vi "cook.vi"(8 "error in (no error)":errorcluster, 11 "Barbecue in":refnum<class "Barbecue.lvclass">) -> (0 "error out":errorcluster, 3 "Barbecue out":refnum<class "Barbecue.lvclass">)   [LabVIEW 2011, in "CookBehaviors.lvlib" / "Barbecue.lvclass"]
uses:
  Barbecue.lvclass
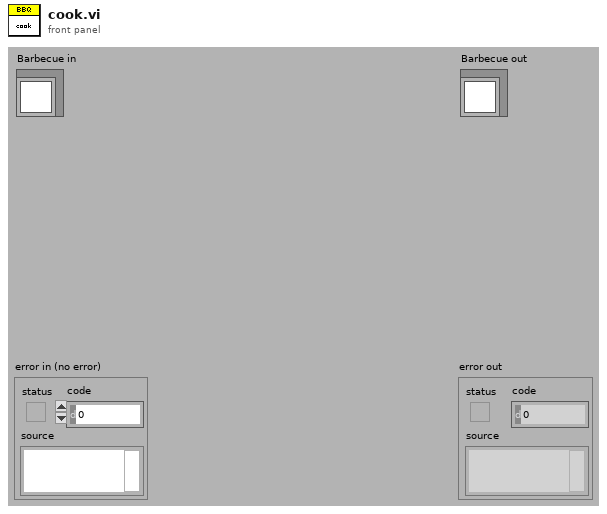
[diagram p1: front panel]
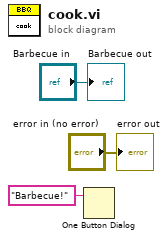
[diagram p0: block diagram]
diagram:
  n1 = One Button Dialog(message="Barbecue!") -> ()  [unwired: 1 in, 1 out]
  "error out" <- "error in (no error)"
  "Barbecue out" <- "Barbecue in"
